vi "Create.vi"(8 "error in (no error)":errorcluster, 10 "Input":string) -> (0 "error out":errorcluster, 1 "Cols":i32, 2 "Rows":i32, 3 "Proto":refnum<class "Maze.lvclass">)   [LabVIEW 2021, in "Maze.lvclass"]
uses:
  Maze.lvclass
  Beam/Beam.lvclass
  Maze.lvclass/Maze.ctl
  Helpers/Helpers.lvlib
panel:
  out "Array":string[][](array[string])
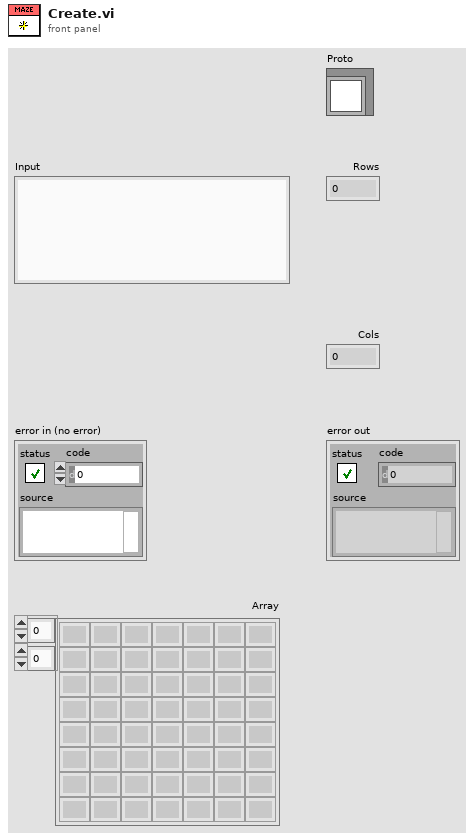
[diagram p1: front panel]
types:
  T1 = map{refnum<class "Beam.lvclass">, refnum<class "Beam.lvclass">[]}
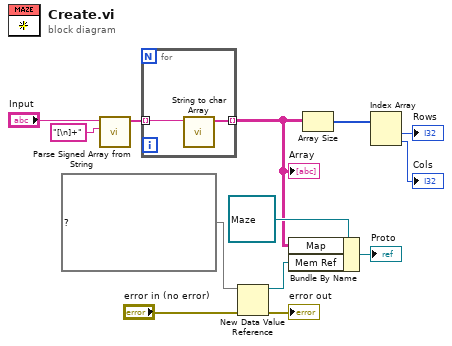
[diagram p0: block diagram]
diagram:
  n1 = call "Parse Signed Array from String.vi"("Delimiter regex"="[\n]+", "Input"="Input") -> ("Parsed Array"=w9:string[])  [unwired: 8 in, 1 out]
  n2 = for {
    tunnel: w9 -> [w15] mode=indexing
    tunnel: [w14] -> w7 mode=indexing
    n3 = call "String to char Array.vi"("Row"=w15) -> ("Array"=w14:string[])  [unwired: 10 in]
  }
  "Array" <- w7
  n4 = New Data Value Reference(data value=T1 {} ("Mem"), error in="error in (no error)") -> (data value reference=w1:refnum<data-value>, error out=→"error out":errorcluster)
  n5 = Bundle By Name(cluster=refnum<class "Maze.lvclass"> refnum ("Proto"), "Map"=w7, "Mem Ref"=w1) -> (→"Proto":refnum<class "Maze.lvclass">)
  n6 = Array Size(array=w7) -> (size(s)=w6:i32[])
  n7 = Index Array(array=w6) -> (element #1=→"Rows":i32, element #2=→"Cols":i32)  [unwired: 2 in]
